vi "tmp_toml_lock_acquire.vi"(8 "error in (no error)":errorcluster, 11 "path in":path) -> (0 "error out":errorcluster, 1 "resolved path":path, 2 "cnt":u8, 3 "lock":refnum<queue>)   [LabVIEW 2017]
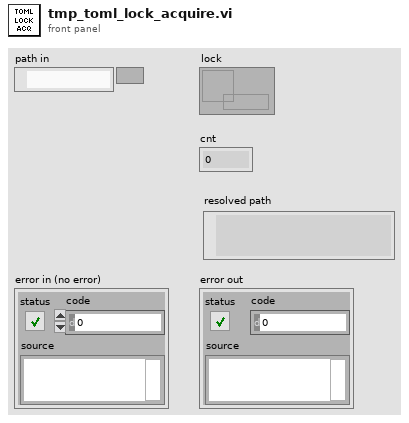
[diagram p1: front panel]
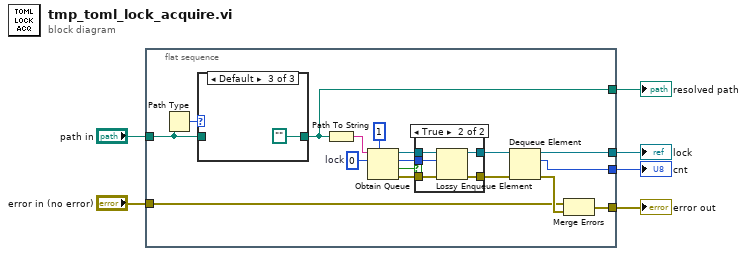
[diagram p0: block diagram]
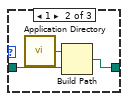
[diagram p4: hidden frame]
diagram:
  n1 = flat-sequence {
    tunnel: "path in" -> [w22]
    tunnel: [w20] -> w5
    tunnel: [w19] -> w4
    tunnel: [w9] -> w3
    tunnel: "error in (no error)" -> [w8]
    tunnel: [w7] -> w1
    frame #0 {
      w13 = u8 0  # lock
      n2 = Path Type(1:w22) -> (0:w21:i16)
      n3 = case shown="Default" w21 {
        tunnel: w22 -> [w30 w32 _]
        tunnel: [w30 w31 path ""] -> w7
        frame 0 {
        }
        frame 1 {
          n4 = call <vilib>:"Application Directory.vi"() -> ("Application Directory"=w33:path)
          n5 = Build Path(base path=w33, name or relative path=w32) -> (appended path=w31:path)
        }
        frame Default {
        }
      }
      n6 = Path To String(path=w7) -> (string=w10:string)
      n7 = Obtain Queue(max queue size (-1, unlimited)=1, name (unnamed)=w10, element data type=w13) -> (queue out=w12:refnum<queue>, created new?=w15:bool, error out=w14:errorcluster)  [unwired: 2 in]
      n8 = case shown="True" w15 {
        tunnel: w12 -> [w24 w29]
        tunnel: w13 -> [_ w28]
        tunnel: w14 -> [w23 w27]
        tunnel: [w24 w26] -> w16
        tunnel: [w23 w25] -> w17
        frame False {
        }
        frame True {
          n9 = Lossy Enqueue Element(queue=w29, element=w28, error in (no error)=w27) -> (queue out=w26:refnum<queue>, error out=w25:errorcluster)  [unwired: 2 out]
        }
      }
      n10 = Dequeue Element(queue=w16, error in (no error)=w17) -> (queue out=w19:refnum<queue>, element=w20:u8, error out=w18:errorcluster)  [unwired: 1 in, 1 out]
      n11 = Merge Errors(w8, w18) -> (w9:errorcluster)
    }
  }
  "cnt" <- w5
  "lock" <- w4
  "error out" <- w3
  "resolved path" <- w1
